vi "Pre Launch Init.vi"(11 "Signal_Gen in":refnum<class "Signal_Gen.lvclass">) -> (0 "error out":errorcluster, 3 "Signal_Gen out":refnum<class "Signal_Gen.lvclass">)   [LabVIEW 2019, in "Signal_Gen.lvlib" / "Signal_Gen.lvclass"]
doc: "(<B>Filename</B>: Actor Framework.lvlib:Actor.lvclass:Pre Launch Init.vi)\n\nDefines behavior that occurs after the Launch Nested Actor method is invoked but before the actor's Actor Core method begins running.\n\nBy default, this method does nothing. A descendant class may override it to define behavior."
uses:
  Signal_Gen.lvclass
  Signal_Gen.lvclass/Signal_Gen.ctl
  <vilib>/ActorFramework/Actor/Actor.lvclass
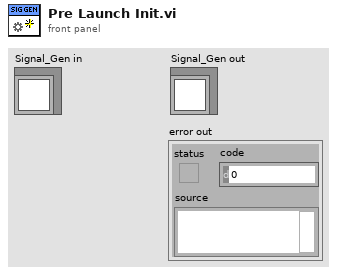
[diagram p1: front panel]
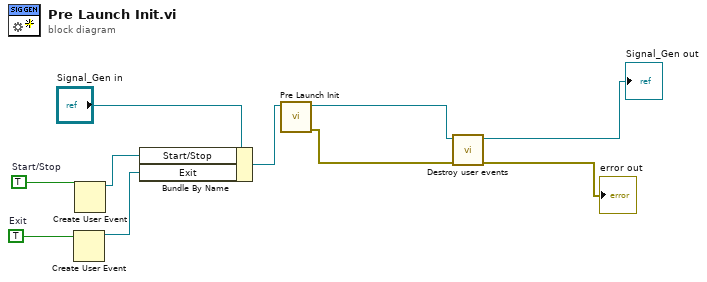
[diagram p0: block diagram]
diagram:
  w8 = TRUE  # Exit
  w9 = TRUE  # Start/Stop
  n1 = Create User Event(user event datatype=w8) -> (user event=w5:refnum<user-event>)  [unwired: 1 in, 1 out]
  n2 = Create User Event(user event datatype=w9) -> (user event=w6:refnum<user-event>)  [unwired: 1 in, 1 out]
  n3 = Bundle By Name(cluster="Signal_Gen in", "Start/Stop"=w6, "Exit"=w5) -> (w7:refnum<class "Signal_Gen.lvclass">)
  n4 = call-parent "Pre Launch Init.vi"("Actor in"=w7) -> ("error out"=w4:errorcluster, "Actor out"=w1:refnum<class "Signal_Gen.lvclass">)  [unwired: 9 in]
  n5 = call "Destroy user events.vi"("error in (no error)"=w4, "Signal_Gen in"=w1) -> ("error out"=→"error out":errorcluster, "Signal_Gen out"=→"Signal_Gen out":refnum<class "Signal_Gen.lvclass">)  [unwired: 8 in]
